vi "ESP32_Socket_NoLoop_MulitpleCmd.vi"() -> ()   [LabVIEW 2022 SP3]
doc: "Demonstrates how to open a connection to an TCP server, read the data being sent, and display the data on a chart. This VI is designed to stop if the TCP connection is terminated."
panel:
  out "new picture":picture
  in  "Image Path":path
  in  "Stop":bool
  in  "Server Closed 2":string="The server VI closed the connection."
  in  "IP Address":string="10.0.0.127"
  out "Response":string
  in  "Stop Driving":bool
  in  "Right":bool
  in  "Left":bool
  in  "Backward":bool
  in  "Forward":bool
  in  "Track 2":bool
  in  "Track 1":bool
  # "Track Selection"
  # "LiDAR Clustered Point Clouds"
  # "Manual Override"
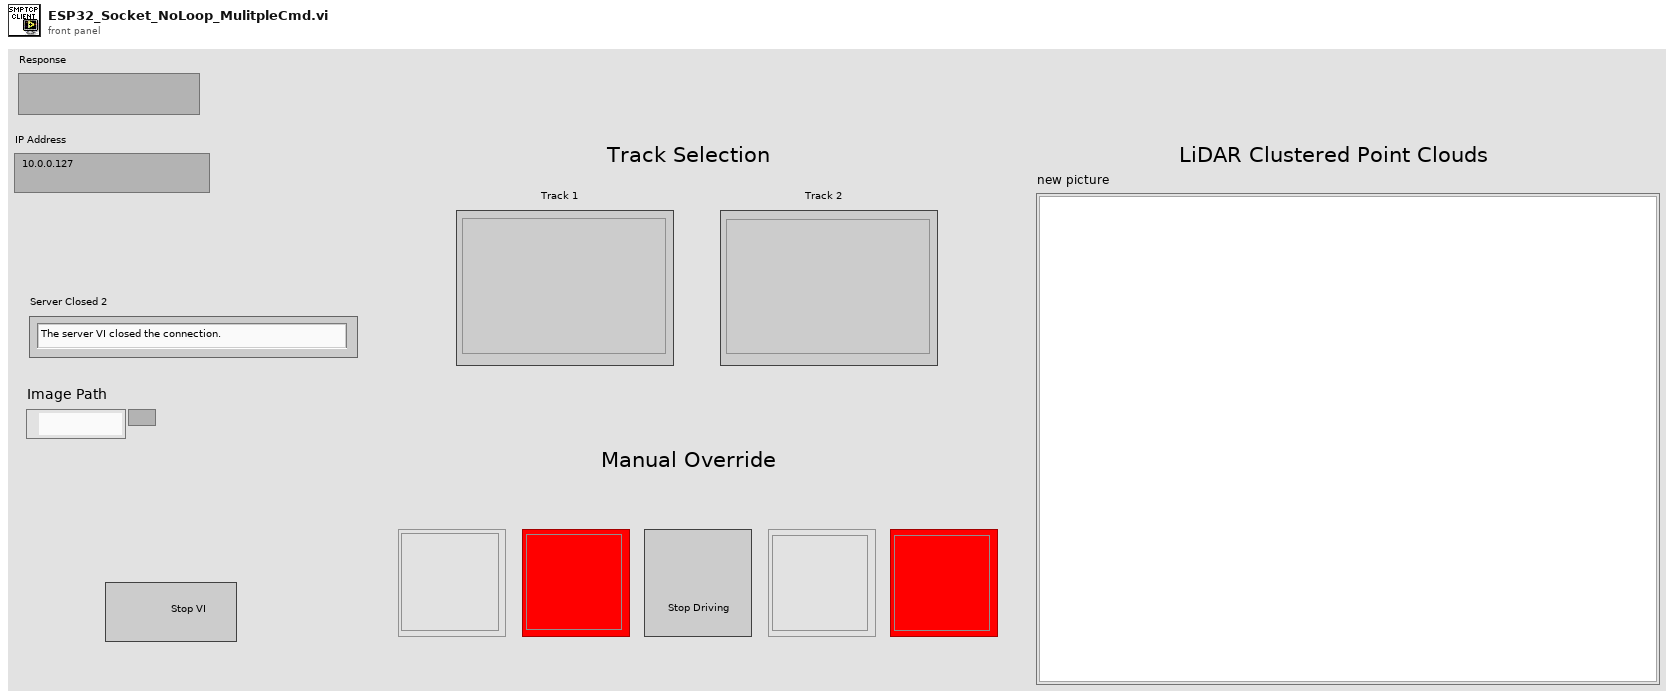
[diagram p1: front panel]
types:
  T1 = enum16{"Standard", "Buffered", "CRLF", "Immediate"}
  T2 = typedef "imagedata.ctl" = cluster{"image type":i32, "image depth":i32, "image":u8[], "mask":u8[], "colors":u32[], "Rectangle":cluster{"left":i16, "top":i16, "right":i16, "bottom":i16}}
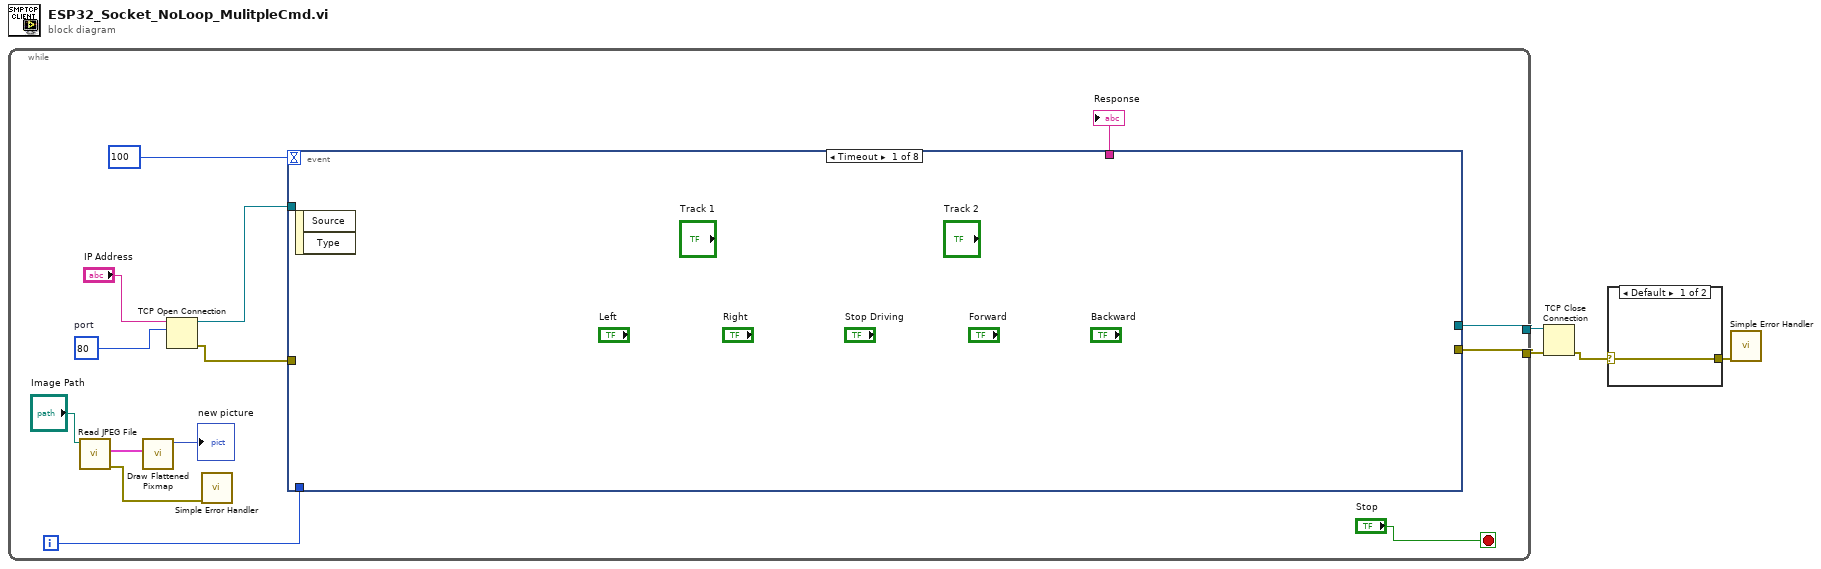
[diagram p0: block diagram]
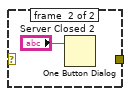
[diagram p2: hidden frame]
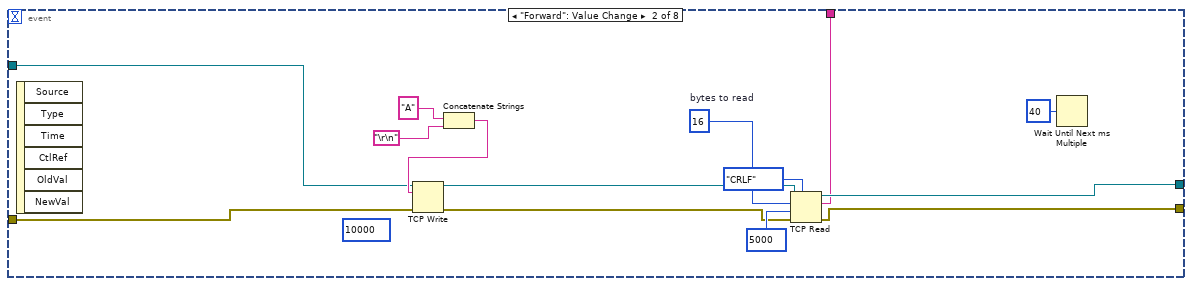
[diagram p3: hidden frame]
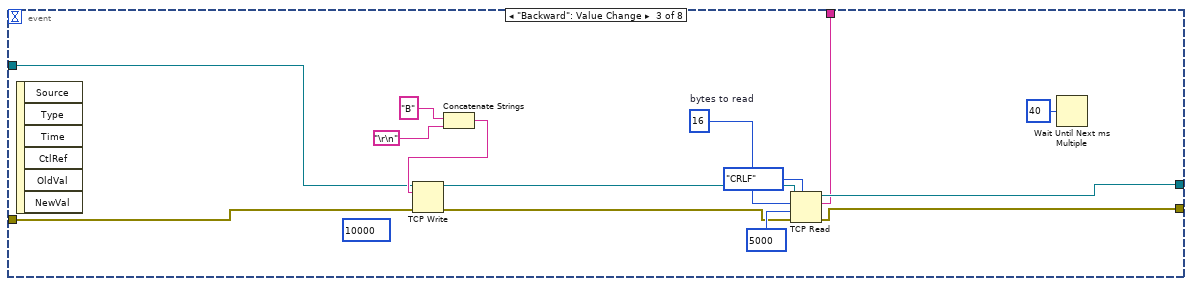
[diagram p4: hidden frame]
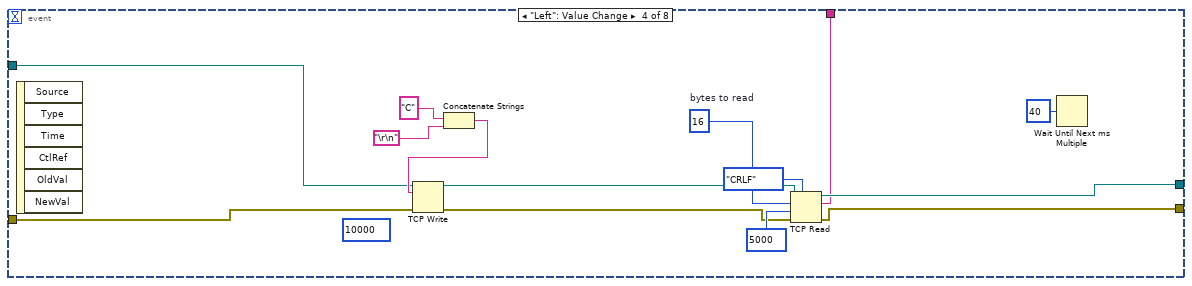
[diagram p5: hidden frame]
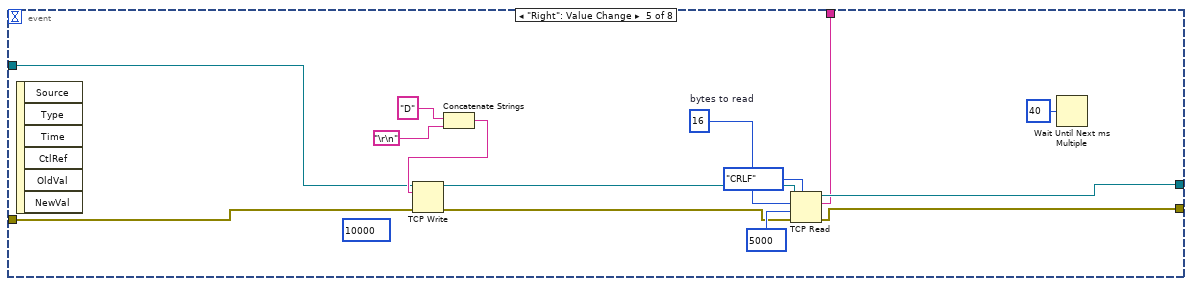
[diagram p6: hidden frame]
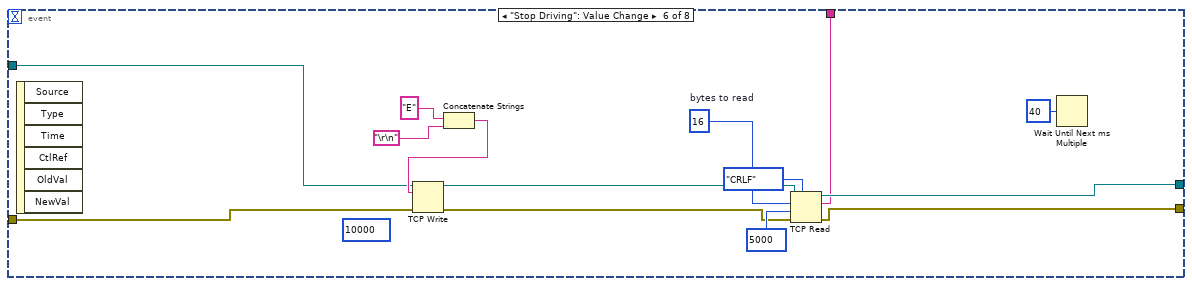
[diagram p7: hidden frame]
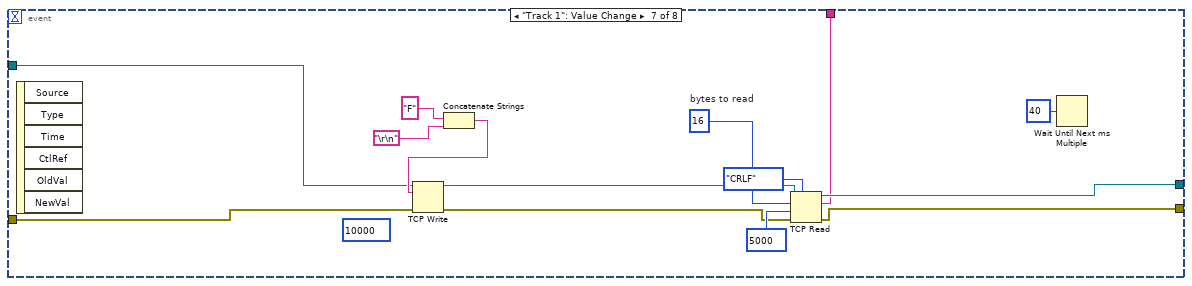
[diagram p8: hidden frame]
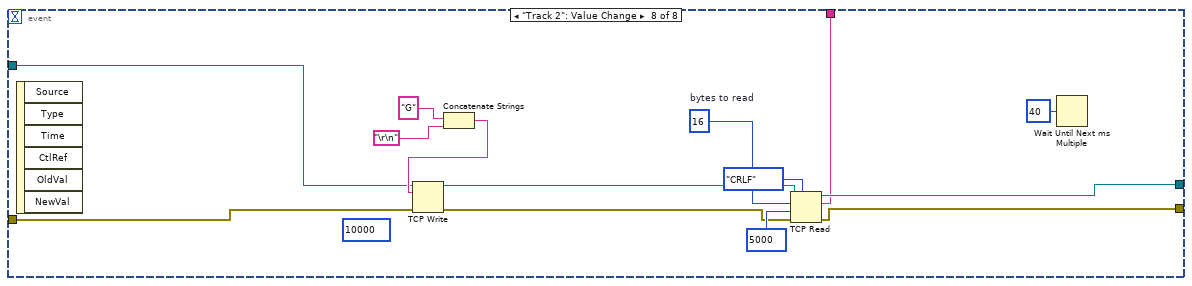
[diagram p9: hidden frame]
diagram:
  n1 = while {
    tunnel: [w11] -> w2
    tunnel: [w10] -> w1
    i -> [w17]
    stop <- "Stop" stop-if-true
    w14 = u16 80  # port
    n2 = call <vilib>:"Read JPEG File.vi"("path to JPEG file"="Image Path") -> ("error out"=w8:errorcluster, "image data"=w6:T2)  [unwired: 1 in, 8 out]
    n3 = call <vilib>:"Draw Flattened Pixmap.vi"("image data"=w6) -> ("new picture"=→"new picture":picture)  [unwired: 1 in, 7 out]
    n4 = TCP Open Connection(address="IP Address", remote port or service name=w14) -> (connection ID=w12:refnum<k5>, error out=w13:errorcluster)  [unwired: 3 in]
    n5 = call <vilib>:"Simple Error Handler.vi"("error in (no error)"=w8) -> ()  [unwired: 4 in, 5 out]
    n6 = event shown="[0] Timeout" {
      selector: _ -> [_ _ _ _ _ _ _ _]
      dyn-events: _ -> [_ _ _ _ _ _ _ _]
      timeout: 100 -> [_ _ _ _ _ _ _ _]
      tunnel: w17 -> [_ _ _ _ _ _ _ _]
      tunnel: w13 -> [_ w23 w37 w51 w65 w79 w93 w107]
      tunnel: w12 -> [_ w22 w36 w50 w64 w78 w92 w106]
      tunnel: [_ w21 w35 w49 w63 w77 w91 w105] -> w11
      tunnel: [_ w20 w34 w48 w62 w76 w90 w104] -> w10
      tunnel: [_ w19 w33 w47 w61 w75 w89 w103] -> w9
      event Timeout {
        n7 = event-data() -> ()  [unwired: 1 in, 2 out]
      }
      event "Forward": Value Change {
        (unwired) 10000 ("timeout ms (25000)")
        w32 = 16  # bytes to read
        n8 = event-data() -> ()  [unwired: 1 in, 6 out]
        n9 = Concatenate Strings("A" ("data in"), "\r\n") -> (w25:string)
        n10 = TCP Write(connection ID=w22, data in=w25, error in (no error)=w23) -> (connection ID out=w30:refnum<k5>, error out=w24:errorcluster)  [unwired: 1 in, 1 out]
        n11 = TCP Read(connection ID=w30, bytes to read=w32, error in (no error)=w24, 7:T1."CRLF" ("mode (standard)"), 9:5000 ("timeout ms (25000)")) -> (connection ID out=w20:refnum<k5>, data out=w19:string, error out=w21:errorcluster)
        n12 = Wait Until Next ms Multiple(millisecond multiple=u32 40) -> ()  [unwired: 1 out]
      }
      event "Backward": Value Change {
        (unwired) 10000 ("timeout ms (25000)")
        w46 = 16  # bytes to read
        n13 = event-data() -> ()  [unwired: 1 in, 6 out]
        n14 = Concatenate Strings("B" ("data in"), "\r\n") -> (w39:string)
        n15 = TCP Write(connection ID=w36, data in=w39, error in (no error)=w37) -> (connection ID out=w44:refnum<k5>, error out=w38:errorcluster)  [unwired: 1 in, 1 out]
        n16 = TCP Read(connection ID=w44, bytes to read=w46, error in (no error)=w38, 7:T1."CRLF" ("mode (standard)"), 9:5000 ("timeout ms (25000)")) -> (connection ID out=w34:refnum<k5>, data out=w33:string, error out=w35:errorcluster)
        n17 = Wait Until Next ms Multiple(millisecond multiple=u32 40) -> ()  [unwired: 1 out]
      }
      event "Left": Value Change {
        (unwired) 10000 ("timeout ms (25000)")
        w60 = 16  # bytes to read
        n18 = event-data() -> ()  [unwired: 1 in, 6 out]
        n19 = Concatenate Strings("C" ("data in"), "\r\n") -> (w53:string)
        n20 = TCP Write(connection ID=w50, data in=w53, error in (no error)=w51) -> (connection ID out=w58:refnum<k5>, error out=w52:errorcluster)  [unwired: 1 in, 1 out]
        n21 = TCP Read(connection ID=w58, bytes to read=w60, error in (no error)=w52, 7:T1."CRLF" ("mode (standard)"), 9:5000 ("timeout ms (25000)")) -> (connection ID out=w48:refnum<k5>, data out=w47:string, error out=w49:errorcluster)
        n22 = Wait Until Next ms Multiple(millisecond multiple=u32 40) -> ()  [unwired: 1 out]
      }
      event "Right": Value Change {
        (unwired) 10000 ("timeout ms (25000)")
        w74 = 16  # bytes to read
        n23 = event-data() -> ()  [unwired: 1 in, 6 out]
        n24 = Concatenate Strings("D" ("data in"), "\r\n") -> (w67:string)
        n25 = TCP Write(connection ID=w64, data in=w67, error in (no error)=w65) -> (connection ID out=w72:refnum<k5>, error out=w66:errorcluster)  [unwired: 1 in, 1 out]
        n26 = TCP Read(connection ID=w72, bytes to read=w74, error in (no error)=w66, 7:T1."CRLF" ("mode (standard)"), 9:5000 ("timeout ms (25000)")) -> (connection ID out=w62:refnum<k5>, data out=w61:string, error out=w63:errorcluster)
        n27 = Wait Until Next ms Multiple(millisecond multiple=u32 40) -> ()  [unwired: 1 out]
      }
      event "Stop Driving": Value Change {
        (unwired) 10000 ("timeout ms (25000)")
        w88 = 16  # bytes to read
        n28 = event-data() -> ()  [unwired: 1 in, 6 out]
        n29 = Concatenate Strings("E" ("data in"), "\r\n") -> (w81:string)
        n30 = TCP Write(connection ID=w78, data in=w81, error in (no error)=w79) -> (connection ID out=w86:refnum<k5>, error out=w80:errorcluster)  [unwired: 1 in, 1 out]
        n31 = TCP Read(connection ID=w86, bytes to read=w88, error in (no error)=w80, 7:T1."CRLF" ("mode (standard)"), 9:5000 ("timeout ms (25000)")) -> (connection ID out=w76:refnum<k5>, data out=w75:string, error out=w77:errorcluster)
        n32 = Wait Until Next ms Multiple(millisecond multiple=u32 40) -> ()  [unwired: 1 out]
      }
      event "Track 1": Value Change {
        (unwired) 10000 ("timeout ms (25000)")
        w102 = 16  # bytes to read
        n33 = event-data() -> ()  [unwired: 1 in, 6 out]
        n34 = Concatenate Strings("F" ("data in"), "\r\n") -> (w95:string)
        n35 = TCP Write(connection ID=w92, data in=w95, error in (no error)=w93) -> (connection ID out=w100:refnum<k5>, error out=w94:errorcluster)  [unwired: 1 in, 1 out]
        n36 = TCP Read(connection ID=w100, bytes to read=w102, error in (no error)=w94, 7:T1."CRLF" ("mode (standard)"), 9:5000 ("timeout ms (25000)")) -> (connection ID out=w90:refnum<k5>, data out=w89:string, error out=w91:errorcluster)
        n37 = Wait Until Next ms Multiple(millisecond multiple=u32 40) -> ()  [unwired: 1 out]
      }
      event "Track 2": Value Change {
        (unwired) 10000 ("timeout ms (25000)")
        w116 = 16  # bytes to read
        n38 = event-data() -> ()  [unwired: 1 in, 6 out]
        n39 = Concatenate Strings("G" ("data in"), "\r\n") -> (w109:string)
        n40 = TCP Write(connection ID=w106, data in=w109, error in (no error)=w107) -> (connection ID out=w114:refnum<k5>, error out=w108:errorcluster)  [unwired: 1 in, 1 out]
        n41 = TCP Read(connection ID=w114, bytes to read=w116, error in (no error)=w108, 7:T1."CRLF" ("mode (standard)"), 9:5000 ("timeout ms (25000)")) -> (connection ID out=w104:refnum<k5>, data out=w103:string, error out=w105:errorcluster)
        n42 = Wait Until Next ms Multiple(millisecond multiple=u32 40) -> ()  [unwired: 1 out]
      }
    }
    "Response" <- w9
  }
  n43 = TCP Close Connection(connection ID=w1, error in (no error)=w2) -> (error out=w3:errorcluster)  [unwired: 1 in, 1 out]
  n44 = case shown="Default" w3 {
    selector: w3 -> [w117 _]
    tunnel: [w117 _] -> w4
    frame #0 {
    }
    frame #1 {
      n45 = One Button Dialog(message="Server Closed 2") -> ()  [unwired: 1 in, 1 out]
    }
  }
  n46 = call <vilib>:"Simple Error Handler.vi"("error in (no error)"=w4) -> ()  [unwired: 4 in, 5 out]
